vi "Setpoint calculation.vi"(9 "PWM Range":cluster{"High PW":dbl, "Low PW":dbl}={"High PW"=5.8, "Low PW"=5.0}, 10 "Test Variables":T1={"Setpoint Function"=enum."Ramp", "Max Diam (mm)"=70.0, "Delay (sec)"=2.0, "T (sec)"=10.0, "Diastole (V)"=0.2, "Systole (V)"=0.5, "Inc Step (s)"=70.0}, 11 "Current test time":dbl) -> (2 "Stop?":bool, 3 "setpoint":dbl)   [LabVIEW 2020]
uses:
  Controls/Test Variables.ctl
  Controls/Serpoint.ctl
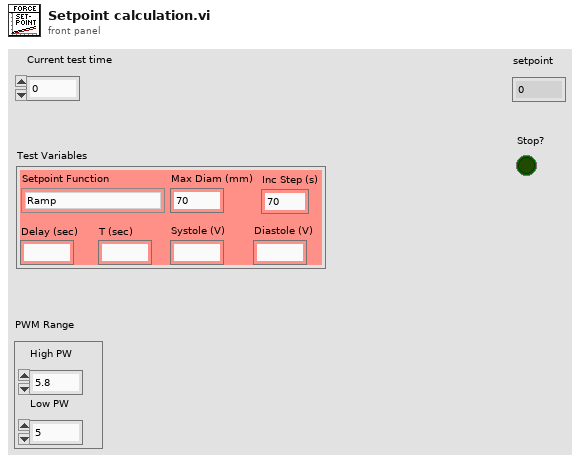
[diagram p1: front panel]
types:
  T1 = typedef "Test Variables.ctl" = cluster{"Setpoint Function":T2, "Max Diam (mm)":dbl, "Delay (sec)":dbl, "T (sec)":dbl, "Diastole (V)":dbl, "Systole (V)":dbl, "Inc Step (s)":dbl}
  T2 = typedef "Serpoint.ctl" = enum16{"Incremental PWM Step", "PWM Step", "Ramp", "Sinusoidal", "Blood-Pressure"}
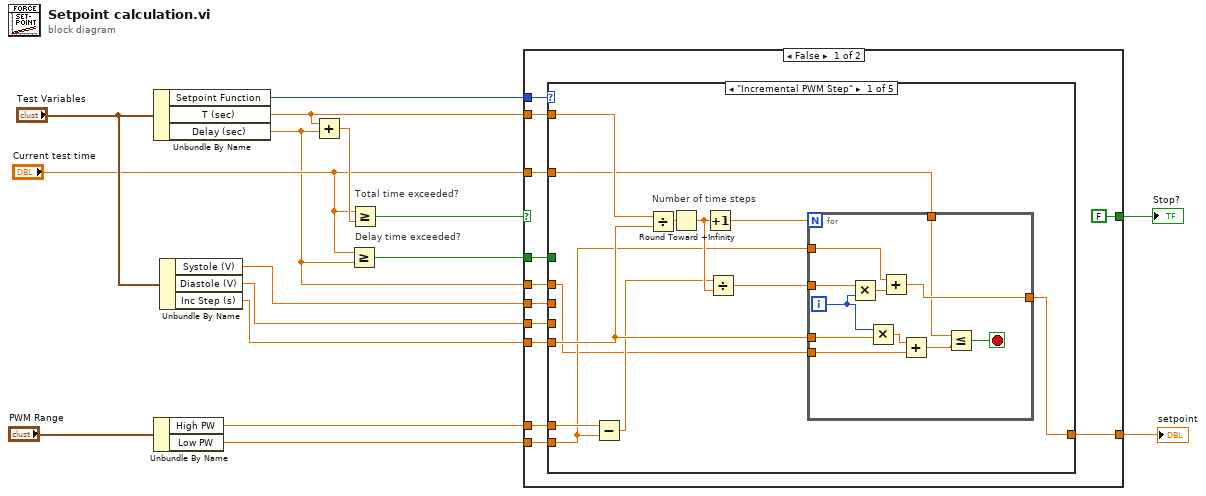
[diagram p0: block diagram]
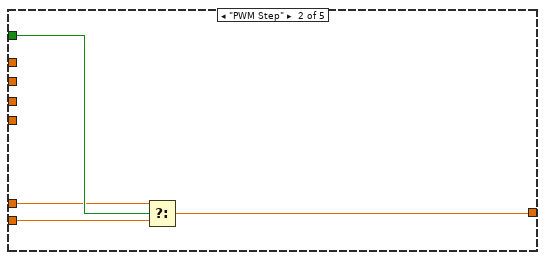
[diagram p2: hidden frame]
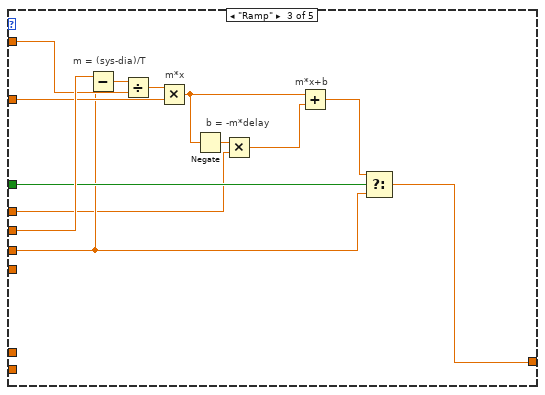
[diagram p3: hidden frame]
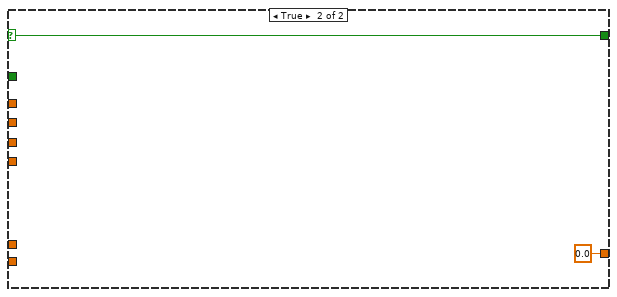
[diagram p6: hidden frame]
diagram:
  # "Delay time exceeded?"
  # "Total time exceeded?"
  n1 = Unbundle By Name("Test Variables") -> ("Setpoint Function"=w16:T2, "T (sec)"=w4:dbl, "Delay (sec)"=w3:dbl)
  n2 = Unbundle By Name("PWM Range") -> ("High PW"=w9:dbl, "Low PW"=w8:dbl)
  n3 = Unbundle By Name("Test Variables") -> ("Systole (V)"=w2:dbl, "Diastole (V)"=w1:dbl, "Inc Step (s)"=w5:dbl)
  n4 = Add(x=w4, y=w3) -> (x+y=w13:dbl)
  n5 = Greater Or Equal?(x="Current test time", y=w3) -> (x >= y?=w11:bool)
  n6 = Greater Or Equal?(x="Current test time", y=w13) -> (x >= y?=w12:bool)
  n7 = case shown="False" w12 {
    selector: w12 -> [_ w72]
    tunnel: w16 -> [w28 _]
    tunnel: w11 -> [w26 _]
    tunnel: "Current test time" -> [w27 _]
    tunnel: w9 -> [w25 _]
    tunnel: w8 -> [w24 _]
    tunnel: [w23 0.0 ("Low PW")] -> w7
    tunnel: [FALSE w72] -> w6
    tunnel: w5 -> [w21 _]
    tunnel: w4 -> [w20 _]
    tunnel: w3 -> [w19 _]
    tunnel: w2 -> [w18 _]
    tunnel: w1 -> [w17 _]
    frame False {
      n8 = case shown="\"Incremental PWM Step\"" w28 {
        tunnel: w27 -> [w30 _ w64 _ _]
        tunnel: w26 -> [_ w55 w63 _ _]
        tunnel: w25 -> [w34 w54 _ _ _]
        tunnel: w24 -> [w33 w53 _ _ _]
        tunnel: [w29 w52 w61 w69 w70] -> w23
        tunnel: w21 -> [w36 _ _ _ _]
        tunnel: w20 -> [w35 _ w66 _ _]
        tunnel: w19 -> [w31 _ w57 _ _]
        tunnel: w18 -> [_ _ w68 _ _]
        tunnel: w17 -> [_ _ w62 w69 w70]
        frame "Incremental PWM Step" {
          # "Number of time steps"
          n9 = Subtract(x=w34, y=w33) -> (x-y=w32:dbl)
          n10 = Divide(x=w35, y=w36) -> (x/y=w40:dbl)
          n11 = Round Toward +Infinity(x=w40) -> (ceil(x): smallest int >= x=w39:dbl)
          n12 = Increment(x=w39) -> (x+1=w38:dbl)
          n13 = Divide(x=w32, y=w39) -> (x/y=w37:dbl)
          n14 = for {
            N: w38 -> [_]
            tunnel: w36 -> [w48]
            tunnel: [w45] -> w29
            tunnel: w37 -> [w44]
            tunnel: w33 -> [w43]
            tunnel: w31 -> [w42]
            tunnel: w30 -> [w41]
            i -> [w46]
            stop <- w49 stop-if-true
            n15 = Multiply(x=w44, y=w46) -> (x*y=w47:dbl)
            n16 = Multiply(x=w46, y=w48) -> (x*y=w51:dbl)
            n17 = Add(x=w43, y=w47) -> (x+y=w45:dbl)
            n18 = Add(x=w51, y=w42) -> (x+y=w50:dbl)
            n19 = Less Or Equal?(x=w41, y=w50) -> (x <= y?=w49:bool)
          }
        }
        frame "PWM Step" {
          n20 = Select(t=w54, s=w55, f=w53) -> (s? t:f=w52:dbl)
        }
        frame "Ramp" {
          # "b = -m*delay"
          # "m*x+b"
          # "m*x"
          # "m = (sys-dia)/T"
          n21 = Subtract(x=w68, y=w62) -> (x-y=w67:dbl)
          n22 = Divide(x=w67, y=w66) -> (x/y=w65:dbl)
          n23 = Multiply(x=w65, y=w64) -> (x*y=w59:dbl)
          n24 = Negate(x=w59) -> (-x=w58:dbl)
          n25 = Multiply(x=w58, y=w57) -> (x*y=w56:dbl)
          n26 = Add(x=w59, y=w56) -> (x+y=w60:dbl)
          n27 = Select(t=w60, s=w63, f=w62) -> (s? t:f=w61:dbl)
        }
        frame "Sinusoidal" {
          # "Not implemented"
        }
        frame "Blood-Pressure" {
          # "Not implemented"
        }
      }
    }
    frame True {
    }
  }
  "setpoint" <- w7
  "Stop?" <- w6
